vi "PulserSettingsSwitch.vi"(0 "Initilize?":bool, 1 "Pulser Ref":refnum<vi>, 5 "Pulser":T5, 7 "Digitizer Settings in":T1 {"Trigger Settings"."Trig Slope" items=["Positive", "Negative"]; "Trigger Settings"."Level (mV)" format="%.2f"; "Trigger Settings"."Trig Coupling" items=["DC 1 MOhm", "AC 1 MOhm", "DC 50 Ohm", "AC 50 Ohm"]; "Trigger Settings"."Trig Source" items=["Chan 1", "External"]; "Rel Dig Delay" format="%.2f"; "DigTimeOut" format="%.2f"; "Avg Num" min=1; "Offset delay (us)" format="%.2f"; "Additional dig delay (us)" format="%.2f"; "Digitizer delay (us)" format="%.2f"}, 9 "Offset delay (us)":dbl, 11 "Delay Corr?":bool=TRUE, 12 "error in (no error)":errorcluster) -> (4 "Digitizer Settings out":T1 {"Trigger Settings"."Trig Slope" items=["Positive", "Negative"]; "Trigger Settings"."Level (mV)" format="%.2f"; "Trigger Settings"."Trig Coupling" items=["DC 1 MOhm", "AC 1 MOhm", "DC 50 Ohm", "AC 50 Ohm"]; "Trigger Settings"."Trig Source" items=["Chan 1", "External"]; "Rel Dig Delay" format="%.2f"; "DigTimeOut" format="%.2f"; "Avg Num" min=1; "Offset delay (us)" format="%.2f"; "Additional dig delay (us)" format="%.2f"; "Digitizer delay (us)" format="%.2f"}, 14 "error out":errorcluster, 15 "Initialization Failed!!":bool)   [LabVIEW 2022 SP3]
uses:
  pulser.ctl
  Digitizers/-DigitizerRoutines/DigitizerSettings.ctl
  Digitizers/-DigitizerRoutines/Digitizer.ctl
  Digitizers/-DigitizerRoutines/DigConfig.ctl
  Digitizers/-DigitizerRoutines/DigitizerID.ctl
  C:/Windows/System32/ADQAPI_dotNet_helper.dll
  Windows/System32/ADQAPI_dotNet_helper.dll
  PulserGlobals.vi
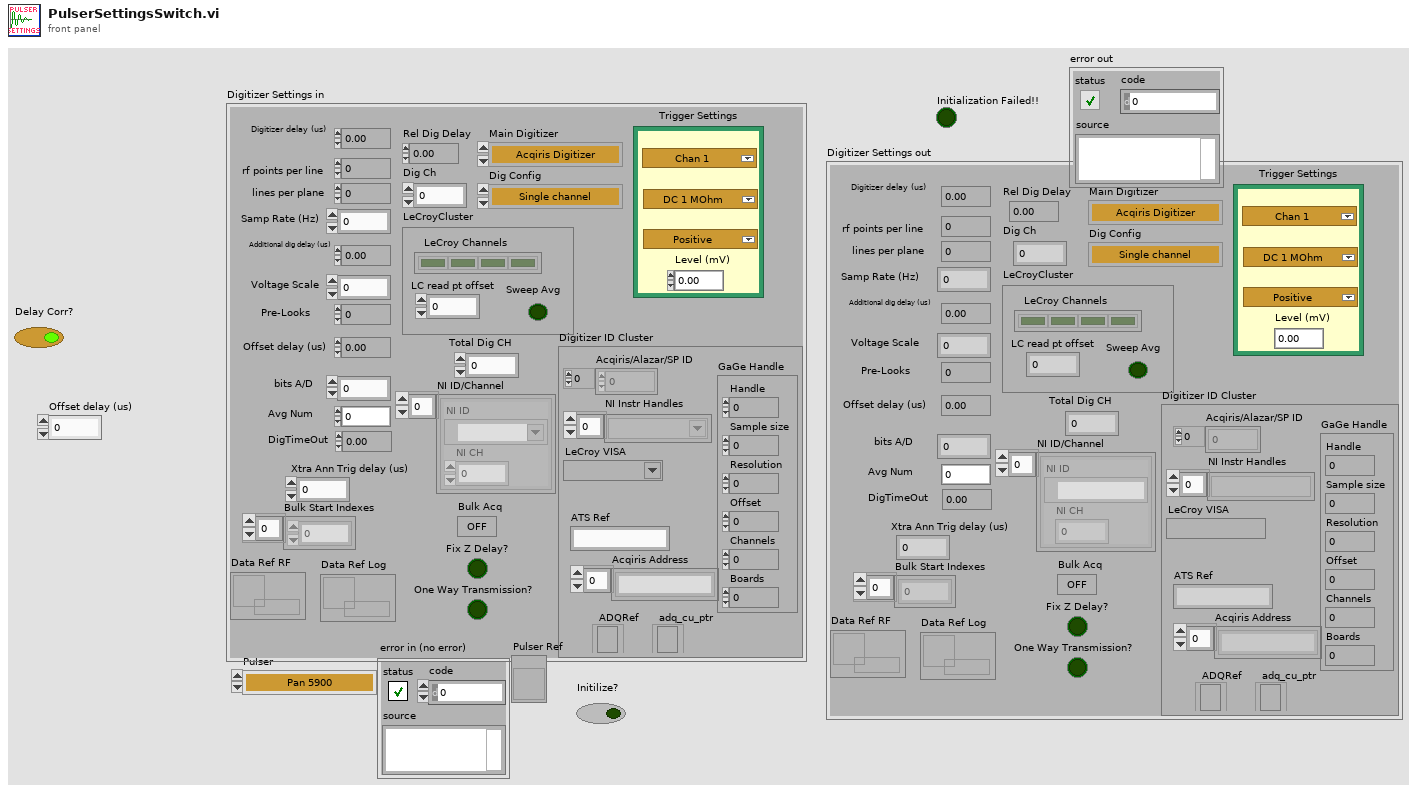
[diagram p1: front panel]
types:
  T1 = typedef "DigitizerSettings.ctl" = cluster{"Digitizer delay (us) ":dbl, "rf points per line":i32, "lines per plane":i32, "Samp Rate (Hz)":dbl, "Additional dig delay (us)":dbl, "Voltage Scale":dbl, "Pre-Looks":i32, "Offset delay (us)":dbl, "bits A/D":i8, "Avg Num":i32, "DigTimeOut":sgl, "Rel Dig Delay":sgl, "Dig Ch":i32, "LeCroyCluster":cluster{"LeCroy Channels":bool[], "LC read pt offset":dbl, "Sweep Avg":bool}, "Main Digitizer":T2, "Dig Config":T3, "Digitizer ID Cluster":T4, "Trigger Settings":cluster{"Trig Source":u16, "Trig Coupling":u16, "Trig Slope":u16, "Level (mV)":dbl}, "Bulk Acq":bool, "Bulk Start Indexes":i32[], "Data Ref RF":refnum<data-value>, "NI ID/Channel":cluster{"NI ID":refnum<k15>, "NI CH":i32}[], "Total Dig CH":i32, "Xtra Ann Trig delay (us)":dbl, "Fix Z Delay?":bool, "One Way Transmission?":bool, "Data Ref Log":refnum<data-value>}
  T2 = typedef "Digitizer.ctl" = enum16{"Acqiris Digitizer", "NI Digitizer", "LeCroy", "GaGe", "AlazarTech", "No Digitizer", "Teledyne"}
  T3 = typedef "DigConfig.ctl" = enum16{"Single channel", "2 Chans w/ 2 Acqiris", "2 Chans w/ 1 Acqiris", "5-CH Pulser New", "5-CH pulser w/ ann array", "5-pass style ann array", "Empty"}
  T4 = typedef "DigitizerID.ctl" = cluster{"Acqiris/Alazar/SP ID":u32[], "NI Instr Handles":refnum<k15>[], "LeCroy VISA":refnum<visa-resource-name>, "GaGe Handle":cluster{"Handle":u32, "Sample size":u32, "Resolution":i32, "Offset":i32, "Channels":u32, "Boards":u32}, "ATS Ref":string, "Acqiris Address":string[], "ADQRef":refnum<k24>, "adq_cu_ptr":refnum<k24>}
  T5 = typedef "pulser.ctl" = enum16{"Pan 5900", "Daxsonics", "Agilent 33xxx", "UTEX", "JSR", "WMC Mono-Cycle", "No Pulser", "NYU AVTECH", "Tabor W1281A", "Pan 5800", "Unlisted", "Tabor WX2182B"}
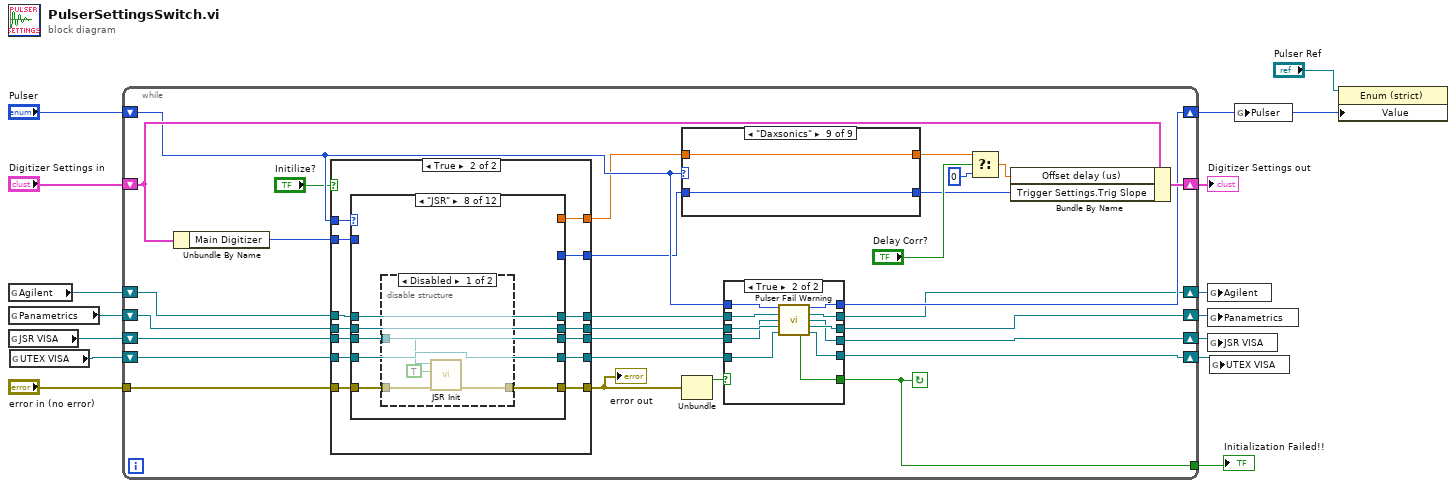
[diagram p0: block diagram]
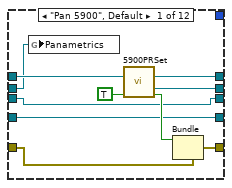
[diagram p3: hidden frame]
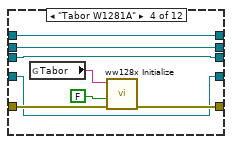
[diagram p6: hidden frame]
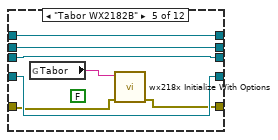
[diagram p7: hidden frame]
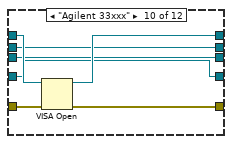
[diagram p12: hidden frame]
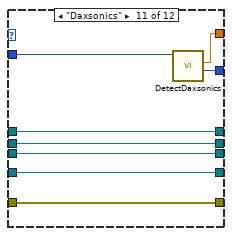
[diagram p13: hidden frame]
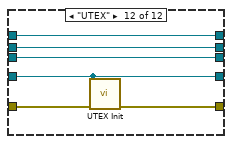
[diagram p14: hidden frame]
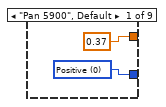
[diagram p15: hidden frame]
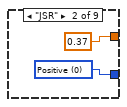
[diagram p16: hidden frame]
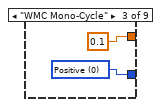
[diagram p17: hidden frame]
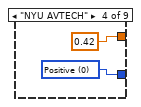
[diagram p18: hidden frame]
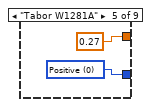
[diagram p19: hidden frame]
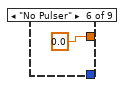
[diagram p20: hidden frame]
diagram:
  n1 = global read "PulserGlobals.vi" "Agilent"() -> (w10:refnum<visa-resource-name>)
  n2 = global read "PulserGlobals.vi" "Panametrics"() -> (w6:refnum<visa-resource-name>)
  n3 = global read "PulserGlobals.vi" "JSR VISA"() -> (w4:refnum<visa-resource-name>)
  n4 = global read "PulserGlobals.vi" "UTEX VISA"() -> (w2:refnum<visa-resource-name>)
  n5 = while {
    shift-right: [w44] -> w14
    shift-left: "Digitizer Settings in" -> [w43]
    shift-right: [w36] -> w8
    shift-left: "Pulser" -> [w31]
    tunnel: "error in (no error)" -> [w39]
    tunnel: [w35] -> w11
    shift-right: [w32] -> w9
    shift-left: w10 -> [w34]
    shift-right: [w25] -> w5
    shift-left: w6 -> [w26]
    shift-right: [w19] -> w3
    shift-left: w4 -> [w21]
    shift-right: [w18] -> w1
    shift-left: w2 -> [w16]
    stop <- w35 continue-if-true
    n6 = Unbundle By Name(w43) -> ("Main Digitizer"=w22:T2)
    n7 = case shown="True" "Initilize?" {
      tunnel: w39 -> [w48 w63]
      tunnel: [w48 w62] -> w38
      tunnel: w34 -> [w49 w61]
      tunnel: [w49 w60] -> w33
      tunnel: w31 -> [_ w59]
      tunnel: [w47 w58] -> w27
      tunnel: w26 -> [w47 w57]
      tunnel: [_ w56] -> w24
      tunnel: [_ w55] -> w23
      tunnel: w22 -> [_ w54]
      tunnel: w21 -> [w46 w53]
      tunnel: [w46 w52] -> w20
      tunnel: [w45 w51] -> w17
      tunnel: w16 -> [w45 w50]
      frame False {
      }
      frame True {
        n8 = case shown="\"JSR\"" w59 {
          tunnel: w63 -> [w72 w77 w82 w88 w91 w102 w107 w111 w122 w126 w137 w139]
          tunnel: [w71 w77 w82 w87 w92 w102 w107 w110 w122 w127 w137 w138] -> w62
          tunnel: w61 -> [w68 w76 w81 w86 w97 w101 w106 w113 w121 w129 w136 w143]
          tunnel: [w68 w76 w81 w86 w97 w101 w106 w113 w121 w128 w136 w143] -> w60
          tunnel: [w67 w75 w80 w85 w96 w100 w105 w112 w120 w125 w135 w142] -> w58
          tunnel: w57 -> [w66 w75 w80 w85 w96 w100 w105 w112 w120 w125 w135 w142]
          tunnel: [_ _ _ _ _ _ _ _ _ _ w134 _] -> w56
          tunnel: [_ _ _ _ _ _ _ _ _ _ w133 _] -> w55
          tunnel: w54 -> [_ _ _ _ _ _ _ _ _ _ w132 _]
          tunnel: w53 -> [w65 w74 w79 w84 w95 w99 w104 w109 w119 w124 w131 w141]
          tunnel: [w65 w74 w79 w84 w95 w99 w104 w109 w119 w124 w131 w141] -> w52
          tunnel: [w64 w73 w78 w83 w94 w98 w103 w108 w118 w123 w130 w140] -> w51
          tunnel: w50 -> [w64 w73 w78 w83 w94 w98 w103 w108 w118 w123 w130 w140]
          frame "Pan 5900", Default {
            n9 = global write "PulserGlobals.vi" "Panametrics"(w66) -> ()
            n10 = call "5900PRSet.vi"("ExitSendCmd"=TRUE) -> ("Panametrics Address"=w67:refnum<visa-resource-name>, "no 5900?"=w69:bool)  [unwired: 12 in, 1 out]
            n11 = Bundle(cluster=w72, "status"=w69) -> (w71:errorcluster)  [unwired: 2 in]
          }
          frame "WMC Mono-Cycle" {
          }
          frame "NYU AVTECH" {
          }
          frame "Tabor W1281A" {
            n12 = global read "PulserGlobals.vi" "Tabor"() -> (w89:string)
            n13 = call <instrlib>:"ww128x Initialize.vi"("error in (no error)"=w88, "reset device (Yes)"=FALSE ("Reset (T: Reset)"), "resource name"=w89) -> ("error out"=w87:errorcluster)  [unwired: 7 in, 1 out]
          }
          frame "Tabor WX2182B" {
            (unwired) FALSE ("Reset (T: Reset)")
            n14 = global read "PulserGlobals.vi" "Tabor"() -> (w93:string)
            n15 = call <instrlib>:"wx218x Initialize With Options.vi"("error in (no error)"=w91, "resource name"=w93) -> ("error out"=w92:errorcluster)  [unwired: 8 in, 1 out]
          }
          frame "Pan 5800" {
          }
          frame "No Pulser" {
          }
          frame "JSR" {
            n16 = disable-structure shown="Disabled" {
              disable-tunnel: w111 -> [w117 _]
              disable-tunnel: [w116 _] -> w110
              disable-tunnel: w109 -> [w115 _]
              frame Disabled {
                n17 = call "JSR Init.vi"("error in (no error)"=w117, "Pulser State (T: ON)"=TRUE, "JSR VISA"=w115) -> ("error out"=w116:errorcluster)  [unwired: 7 in, 1 out]
              }
              frame Enabled {
              }
            }
          }
          frame "Unlisted" {
          }
          frame "Agilent 33xxx" {
            n18 = VISA Open(error in (no error)=w126, VISA resource name=w129) -> (VISA resource name=w128:refnum<visa-resource-name>, error out=w127:errorcluster)  [unwired: 3 in]
          }
          frame "Daxsonics" {
            n19 = call "DetectDaxsonics.vi"("Main Digitizer"=w132) -> ("Trig Slope"=w133:u16, "Offset Delay (us)"=w134:dbl)  [unwired: 9 in]
          }
          frame "UTEX" {
            n20 = call "UTEX Init.vi"("error in (no error)"=w139, "VISA resource name"=w140) -> ("error out"=w138:errorcluster)  [unwired: 8 in, 1 out]
          }
        }
      }
    }
    "error out" <- w38
    n21 = case shown="\"Daxsonics\"" w31 {
      tunnel: [w145 w147 w149 w151 w153 _ _ w157 w158] -> w29
      tunnel: [0.37 ("Offset delay (us)") 0.37 ("Offset delay (us)") 0.1 ("Offset delay (us)") 0.42 ("Offset delay (us)") 0.27 ("Offset delay (us)") 0.0 ("Offset delay (us)") "Offset delay (us)" 0.34 ("Offset delay (us)") w159] -> w30
      tunnel: w24 -> [_ _ _ _ _ _ _ _ w159]
      tunnel: w23 -> [_ _ _ _ _ _ _ _ w158]
      frame "Pan 5900", Default {
        w145 = u16 0 items=["Positive", "Negative"] ("Trig Slope")
      }
      frame "JSR" {
        w147 = u16 0 items=["Positive", "Negative"] ("Trig Slope")
      }
      frame "WMC Mono-Cycle" {
        w149 = u16 0 items=["Positive", "Negative"] ("Trig Slope")
      }
      frame "NYU AVTECH" {
        w151 = u16 0 items=["Positive", "Negative"] ("Trig Slope")
      }
      frame "Tabor W1281A" {
        w153 = u16 0 items=["Positive", "Negative"] ("Trig Slope")
      }
      frame "No Pulser" {
      }
      frame "Unlisted" {
      }
      frame "Agilent 33xxx" {
        w157 = u16 0 items=["Positive", "Negative"] ("Trig Slope")
      }
      frame "Daxsonics" {
      }
    }
    n22 = Unbundle(w38) -> ("status"=w37:bool)  [unwired: 2 out]
    n23 = case shown="True" w37 {
      selector: w37 -> [w165 _]
      tunnel: [w165 w170] -> w35
      tunnel: w31 -> [w164 w176]
      tunnel: [w164 w175] -> w36
      tunnel: w33 -> [w163 w174]
      tunnel: [w163 w173] -> w32
      tunnel: w27 -> [w162 w172]
      tunnel: [w162 w171] -> w25
      tunnel: w20 -> [w161 w169]
      tunnel: [w161 w168] -> w19
      tunnel: [w160 w166] -> w18
      tunnel: w17 -> [w160 w167]
      frame False {
      }
      frame True {
        n24 = call "Pulser Fail Warning.vi"("Pulser"=w176, "Agilent"=w174, "JSR"=w169, "Panametrics"=w172, "UTEX"=w167) -> ("Pulser Out"=w175:T5, "Agilent Out"=w173:refnum<visa-resource-name>, "JSR Out"=w168:refnum<visa-resource-name>, "Panametrics Out"=w171:refnum<visa-resource-name>, "Retry"=w170:bool, "UTEX Out"=w166:refnum<visa-resource-name>)  [unwired: 5 in]
      }
    }
    n25 = Select(t=w30, s="Delay Corr?", f=0) -> (s? t:f=w40:dbl)
    n26 = Bundle By Name(cluster=w43, "Offset delay (us)"=w40, "Trigger Settings.Trig Slope"=w29) -> (w44:T1)
  }
  "Digitizer Settings out" <- w14
  "Initialization Failed!!" <- w11
  n27 = global write "PulserGlobals.vi" "Agilent"(w9) -> ()
  n28 = global write "PulserGlobals.vi" "Panametrics"(w5) -> ()
  n29 = global write "PulserGlobals.vi" "JSR VISA"(w3) -> ()
  n30 = global write "PulserGlobals.vi" "UTEX VISA"(w1) -> ()
  n31 = global write "PulserGlobals.vi" "Pulser"(w8) -> ()
  n32 = property class="Enum (strict)"(reference="Pulser Ref", "Value"=w8) -> ()  [unwired: 1 in, 2 out]
